vi "DrawChessboardTearDropSquare.vi"(0 "Bounds":T2, 1 "Skip":bool, 4 "picture in":picture, 5 "Tear Drop Corner":T1) -> (7 "picture out":picture)   [LabVIEW 2020, in "g_ar_toolkit.feature_detection.lvlib"]
uses:
  g_ar_toolkit.feature_detection.lvlib
  Chessboard Teardrop Corner Type.ctl
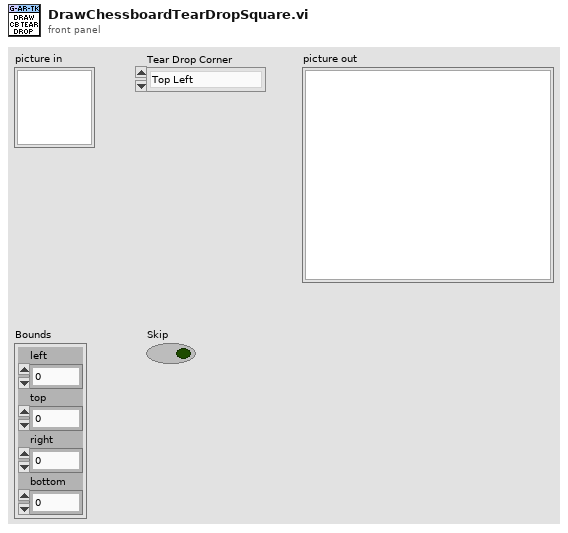
[diagram p1: front panel]
types:
  T1 = typedef "g_ar_toolkit.feature_detection.lvlib/Chessboard Teardrop Corner Type.ctl" = enum16{"Top Left", "Top Right", "Bottom Left", "Bottom Right"}
  T2 = cluster{"left":i16, "top":i16, "right":i16, "bottom":i16}
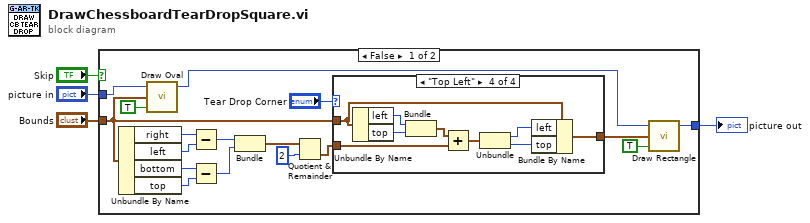
[diagram p0: block diagram]
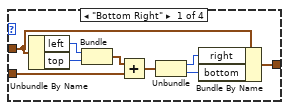
[diagram p2: hidden frame]
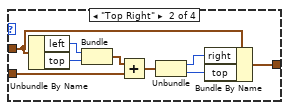
[diagram p3: hidden frame]
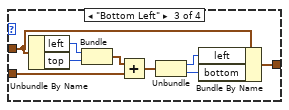
[diagram p4: hidden frame]
diagram:
  n1 = case shown="False" "Skip" {
    tunnel: [w20 w58] -> w4
    tunnel: "picture in" -> [w17 w58]
    tunnel: "Bounds" -> [w7 _]
    frame False {
      n2 = Unbundle By Name(w7) -> ("right"=w16:i16, "left"=w15:i16, "bottom"=w14:i16, "top"=w13:i16)
      n3 = call <vilib>:"Draw Oval.vi"("picture"=w17, "rect"=w7, "fill?(F)"=TRUE) -> ("new picture"=w19:picture)  [unwired: 6 in]
      n4 = Subtract(x=w16, y=w15) -> (x-y=w12:i16)
      n5 = Subtract(x=w14, y=w13) -> (x-y=w11:i16)
      n6 = Bundle(w12, w11) -> (w10:cluster{i16, i16})  [unwired: 1 in]
      n7 = Quotient & Remainder(x=w10, y=i16 2) -> (floor(x/y)=w6:cluster{i16, i16})  [unwired: 1 out]
      n8 = case shown="\"Top Left\"" "Tear Drop Corner" {
        tunnel: w7 -> [w26 w35 w44 w49]
        tunnel: w6 -> [w27 w36 w45 w54]
        tunnel: [w22 w31 w40 w51] -> w5
        frame "Bottom Right" {
          n9 = Unbundle By Name(w26) -> ("left"=w30:i16, "top"=w29:i16)
          n10 = Bundle("left"=w30, "top"=w29) -> (w28:cluster{"left":i16, "top":i16})  [unwired: 1 in]
          n11 = Add(x=w28, y=w27) -> (x+y=w25:cluster{i16, i16})
          n12 = Unbundle(w25) -> (w24:i16, w23:i16)
          n13 = Bundle By Name(cluster=w26, "right"=w24, "bottom"=w23) -> (w22:T2)
        }
        frame "Top Right" {
          n14 = Unbundle By Name(w35) -> ("left"=w39:i16, "top"=w38:i16)
          n15 = Bundle("left"=w39, "top"=w38) -> (w37:cluster{"left":i16, "top":i16})  [unwired: 1 in]
          n16 = Add(x=w37, y=w36) -> (x+y=w34:cluster{i16, i16})
          n17 = Unbundle(w34) -> (w33:i16, w32:i16)
          n18 = Bundle By Name(cluster=w35, "right"=w33, "top"=w32) -> (w31:T2)
        }
        frame "Bottom Left" {
          n19 = Unbundle By Name(w44) -> ("left"=w48:i16, "top"=w47:i16)
          n20 = Bundle("left"=w48, "top"=w47) -> (w46:cluster{"left":i16, "top":i16})  [unwired: 1 in]
          n21 = Add(x=w46, y=w45) -> (x+y=w43:cluster{i16, i16})
          n22 = Unbundle(w43) -> (w42:i16, w41:i16)
          n23 = Bundle By Name(cluster=w44, "left"=w42, "bottom"=w41) -> (w40:T2)
        }
        frame "Top Left" {
          n24 = Unbundle By Name(w49) -> ("left"=w57:i16, "top"=w56:i16)
          n25 = Bundle("left"=w57, "top"=w56) -> (w55:cluster{"left":i16, "top":i16})  [unwired: 1 in]
          n26 = Add(x=w55, y=w54) -> (x+y=w50:cluster{i16, i16})
          n27 = Unbundle(w50) -> (w53:i16, w52:i16)
          n28 = Bundle By Name(cluster=w49, "left"=w53, "top"=w52) -> (w51:T2)
        }
      }
      n29 = call <vilib>:"Draw Rectangle.vi"("picture"=w19, "rect"=w5, "fill?(F)"=TRUE) -> ("new picture"=w20:picture)  [unwired: 6 in]
    }
    frame True {
    }
  }
  "picture out" <- w4
